vi "X轴连续扫描（初稿）.vi"(0 "VISA I":refnum<visa-resource-name>, 3 "X":dbl, 4 "精度":dbl=0.001, 5 "细分设置":dbl=8.0, 6 "等待时间(ms)":u32=40, 7 "pulDDR2Length":u32, 8 "电机急停":bool, 9 "hDevice":i32, 11 "M-length":dbl, 13 "N-length":dbl) -> (14 "VISA O":refnum<visa-resource-name>, 15 "hDevice out":i32, 16 "X":dbl, 17 "强度图行":dbl[](array[numeric]), 18 "时域谱页":dbl[][](array[numeric]), 19 "幅频谱页":dbl[][](array[numeric]))   [LabVIEW 2016]
panel:
  out "大小":i32[](array[numeric])
  out "幅频谱":dbl[](graph)
  out "时域谱":dbl[](graph)
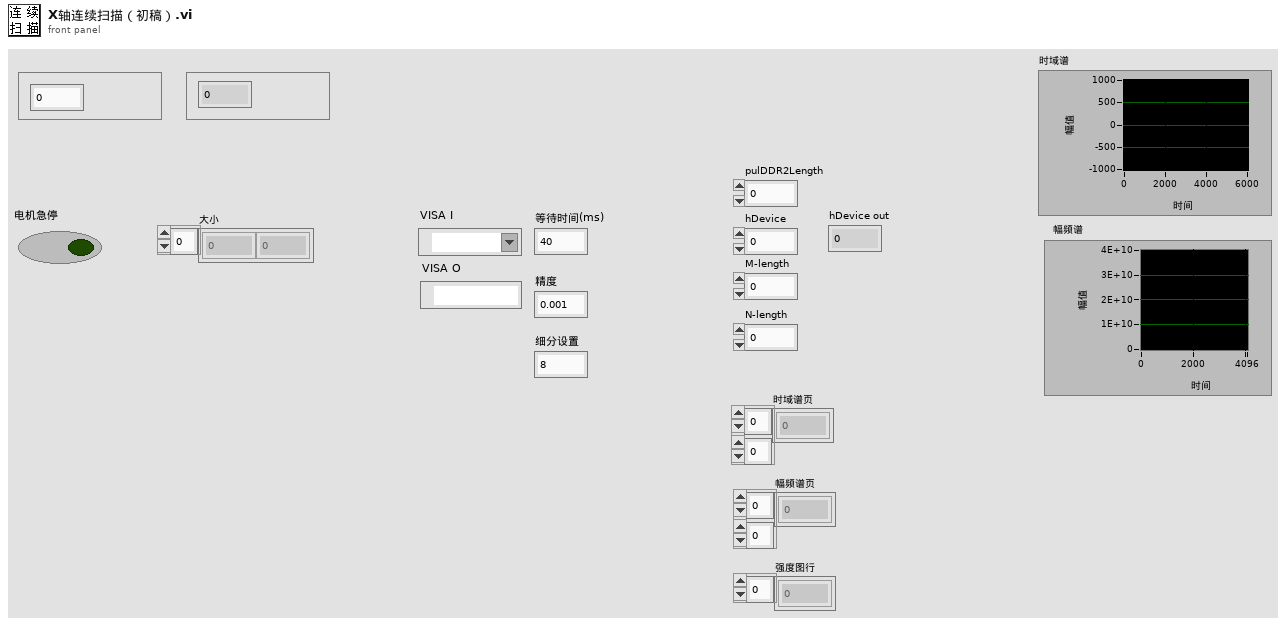
[diagram p1: front panel]
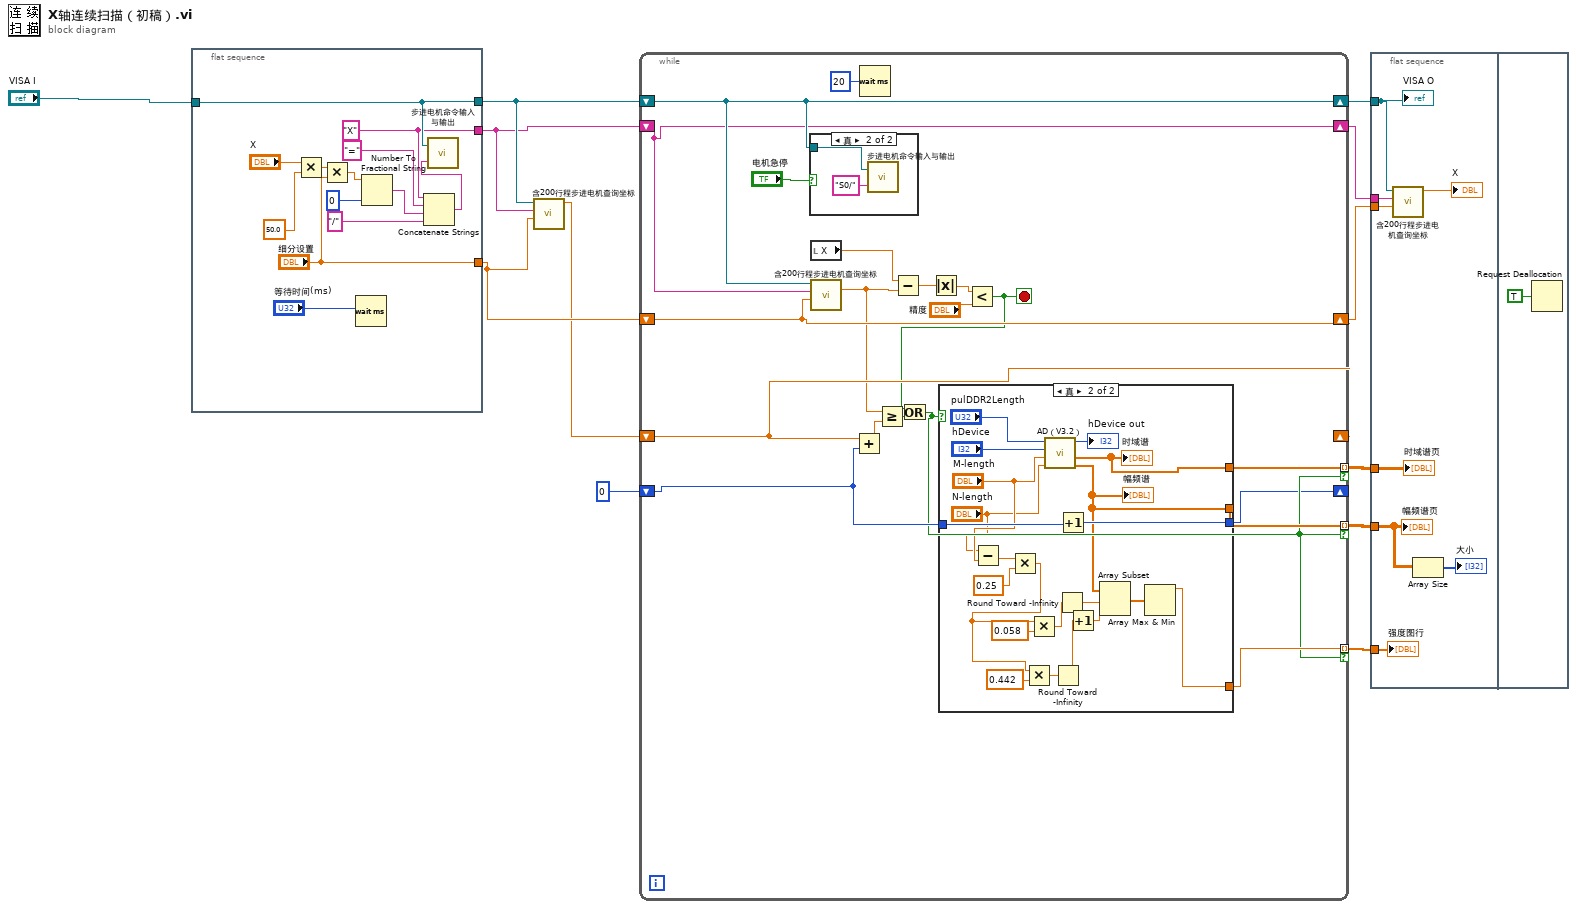
[diagram p0: block diagram]
diagram:
  n1 = flat-sequence {
    tunnel: "VISA I" -> [w17]
    tunnel: [w17] -> w11
    tunnel: ["细分设置"] -> w9
    tunnel: [w14] -> w10
    frame #0 {
      w14 = "X"
      n2 = Multiply(x="X", y=50.0 ("x")) -> (x*y=w20:dbl)
      n3 = Multiply(x=w20, y="细分设置") -> (x*y=w25:dbl)
      n4 = Wait (ms)(milliseconds to wait="等待时间(ms)") -> ()  [unwired: 1 out]
      n5 = Number To Fractional String(number=w25, precision (6)=i16 0 ("精度(6)")) -> (F-format string=w23:string)  [unwired: 2 out]
      n6 = Concatenate Strings(w14, "=" ("字符串"), w23, "/" ("字符串")) -> (w19:string)
      n7 = call "步进电机命令输入与输出.vi"("输入字符串"=w19, "串口通信端口"=w17) -> ()  [unwired: 1 out]
    }
  }
  n8 = call "含200行程步进电机查询坐标.vi"("细分设置"=w9, "查询坐标轴"=w10, "串口通信端口"=w11) -> ("坐标(mm)"=w8:dbl)  [unwired: 8 in]
  n9 = while {
    shift-right: [w43] -> w3
    shift-left: w11 -> [w43]
    shift-right: [w37] -> _
    shift-left: w8 -> [w37]
    shift-right: [w36] -> w1
    shift-left: w9 -> [w36]
    shift-right: [w28] -> w2
    shift-left: w10 -> [w28]
    tunnel: [w35] -> w4 mode=indexing if=w30
    shift-right: [w27] -> _
    shift-left: 0 -> [w34]
    tunnel: [w33] -> w6 mode=indexing if=w30
    tunnel: [w32] -> w5 mode=indexing if=w30
    stop <- w29 stop-if-true
    n10 = case shown="真" "电机急停" {
      tunnel: w43 -> [_ w68]
      frame False {
      }
      frame True {
        n11 = call "步进电机命令输入与输出.vi"("输入字符串"="S0/", "串口通信端口"=w68) -> ()  [unwired: 1 out]
      }
    }
    n12 = local read "X"() -> (w39:dbl)
    n13 = call "含200行程步进电机查询坐标.vi"("细分设置"=w36, "查询坐标轴"=w28, "串口通信端口"=w43) -> ("坐标(mm)"=w26:dbl)  [unwired: 8 in]
    n14 = Add(x=w37, y=w34) -> (x+y=w38:dbl)
    n15 = Wait (ms)(milliseconds to wait=u32 20 ("等待时间（毫秒）")) -> ()  [unwired: 1 out]
    n16 = Greater Or Equal?(x=w26, y=w38) -> (x >= y?=w31:bool)
    n17 = Subtract(x=w39, y=w26) -> (x-y=w45:dbl)
    n18 = Absolute Value(x=w45) -> (abs(x)=w44:dbl)
    n19 = Less?(x=w44, y="精度") -> (x < y?=w29:bool)
    n20 = Or(x=w29, y=w31) -> (x .or. y?=w30:bool)
    n21 = case shown="真" w30 {
      tunnel: [_ w48] -> w35
      tunnel: w34 -> [w46 w64]
      tunnel: [w46 w63] -> w27
      tunnel: [_ w62] -> w33
      tunnel: [_ w47] -> w32
      frame False {
      }
      frame True {
        n22 = Subtract(x="N-length", y="M-length") -> (x-y=w60:dbl)
        n23 = Multiply(x=w60, y=0.25) -> (x*y=w50:dbl)
        n24 = Multiply(x=w50, y=0.442) -> (x*y=w53:dbl)
        n25 = Multiply(x=w50, y=0.058) -> (x*y=w55:dbl)
        n26 = call "AD（V3.2）.vi"("N-length"="N-length", "M-length"="M-length", "hDevice"="hDevice", "pulDDR2Length"="pulDDR2Length") -> ("幅频谱"=w48:dbl[], "时域谱"=w62:dbl[], "hDevice out"=→"hDevice out":i32)  [unwired: 5 in]
        "时域谱" <- w62
        "幅频谱" <- w48
        n27 = Round Toward -Infinity(1:w53) -> (0:w51:dbl)
        n28 = Round Toward -Infinity(1:w55) -> (0:w54:dbl)
        n29 = Increment(x=w64) -> (x+1=w63:i32)
        n30 = Increment(x=w51) -> (x+1=w57:dbl)
        n31 = Array Subset(array=w48, index=w54, length=w57) -> (w49:dbl[])
        n32 = Array Max & Min(array=w49) -> (max value=w47:dbl)  [unwired: 3 out]
      }
    }
  }
  n33 = flat-sequence {
    tunnel: w6 -> [w77]
    tunnel: w5 -> [w76]
    tunnel: w4 -> [w75]
    tunnel: w3 -> [w72]
    tunnel: w2 -> [w71]
    tunnel: w1 -> [w70]
    frame #0 {
      n34 = call "含200行程步进电机查询坐标.vi"("细分设置"=w70, "查询坐标轴"=w71, "串口通信端口"=w72) -> ("坐标(mm)"=→"X":dbl)  [unwired: 8 in]
      n35 = Array Size(array=w75) -> (size(s)=→"大小":i32[])
      "VISA O" <- w72
      "幅频谱页" <- w75
      "时域谱页" <- w77
      "强度图行" <- w76
    }
    frame #1 {
      n36 = Request Deallocation(TRUE ("标志")) -> ()
    }
  }
